vi "Load Env File.vi"(8 "error in (no error)":errorcluster, 11 "Env file path":path=path "C:/batt/test.env") -> (0 "error out":errorcluster, 3 "Variables":variant)   [LabVIEW 2025, in "Battery Prompt.lvlib"]
doc: "Read ENV file and return the environment variables / keys as a variant attributes."
uses:
  <vilib>/Utility/error.llb/Trim Whitespace One-Sided.vi
  Battery Prompt.lvlib
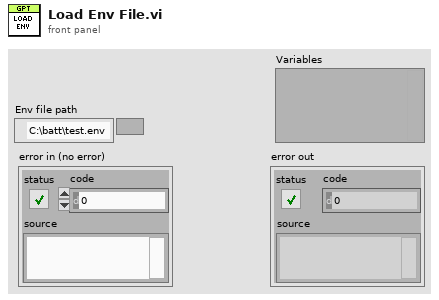
[diagram p1: front panel]
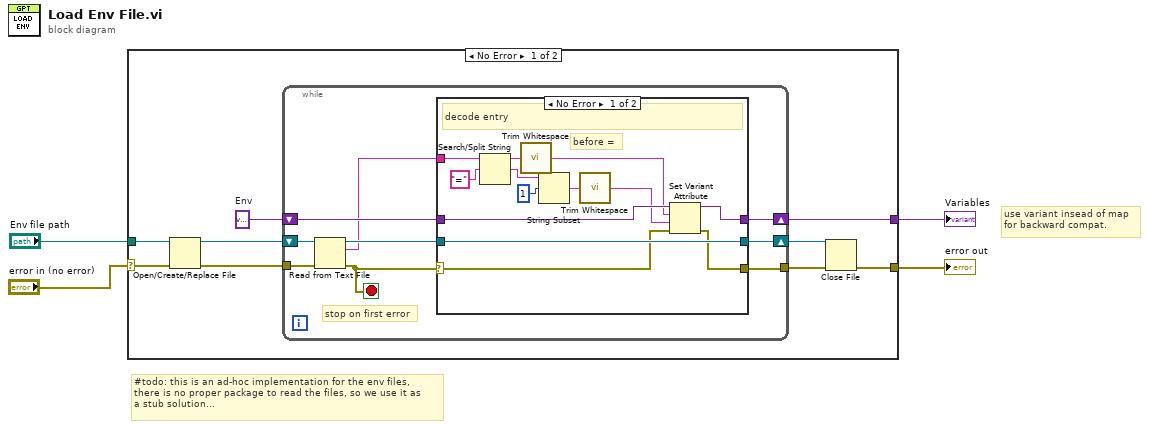
[diagram p0: block diagram]
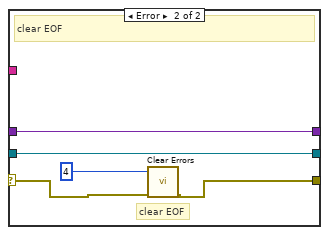
[diagram p2: hidden frame]
diagram:
  # "use variant insead of map\nfor backward compat."
  # "#todo: this is an ad-hoc implementation for the env files,\nthere is no proper package to read the files, so we use it as \na stub solution..."
  n1 = case shown="No Error" "error in (no error)" {
    selector: "error in (no error)" -> [w10 w41]
    tunnel: "Env file path" -> [w12 _]
    tunnel: [w6 w41] -> w2
    tunnel: [w5 _] -> w1
    frame No Error {
      w8 = variant  # Env
      n2 = Open/Create/Replace File(file path (use dialog)=w12, error in=w10) -> (refnum out=w13:refnum<file>, error out=w9:errorcluster)  [unwired: 4 in, 1 out]
      n3 = while {
        shift-right: [w17] -> w11
        shift-left: w13 -> [w22]
        tunnel: w9 -> [w21]
        shift-right: [w15] -> w5
        shift-left: w8 -> [w16]
        tunnel: [w19] -> w7
        stop <- w20 stop-if-true
        # "stop on first error"
        n4 = Read from Text File(file (use dialog)=w22, error in=w21) -> (refnum out=w18:refnum<file>, text=w14:string, error out=w20:errorcluster)  [unwired: 2 in, 1 out]
        n5 = case shown="No Error" w20 {
          selector: w20 -> [w28 w37]
          tunnel: [w27 w36] -> w19
          tunnel: w18 -> [w35 w39]
          tunnel: [w35 w39] -> w17
          tunnel: w16 -> [w26 w40]
          tunnel: [w25 w40] -> w15
          tunnel: w14 -> [w32 _]
          frame No Error {
            # "before ="
            # "decode entry"
            n6 = Search/Split String(string=w32, search string/char (-)="=") -> (substring before match=w34:string, match + rest of string=w31:string)  [unwired: 1 in, 1 out]
            n7 = call <vilib>:"Trim Whitespace.vi"("string"=w34) -> ("trimmed string"=w24:string)  [unwired: 1 in]
            n8 = String Subset(string=w31, offset (0)=1) -> (substring=w29:string)  [unwired: 1 in]
            n9 = call <vilib>:"Trim Whitespace.vi"("string"=w29) -> ("trimmed string"=w23:string)  [unwired: 1 in]
            n10 = Set Variant Attribute(Variant=w26, name=w24, value=w23, error in=w28) -> (Variant out=w25:variant, error out=w27:errorcluster)  [unwired: 1 out]
          }
          frame Error {
            # "clear EOF"
            # "clear EOF"
            n11 = call <vilib>:"Clear Errors.vi"("error in (no error)"=w37, "specific error code to clear (0: all)"=4 ("[error code] (0)")) -> ("error out"=w36:errorcluster)  [unwired: 4 in, 1 out]
          }
        }
      }
      n12 = Close File(refnum=w11, error in=w7) -> (error out=w6:errorcluster)  [unwired: 1 out]
    }
    frame Error {
    }
  }
  "error out" <- w2
  "Variables" <- w1
